vi "trim_space.vi"(1 "string in":string) -> (0 "string out":string)   [LabVIEW 2011]
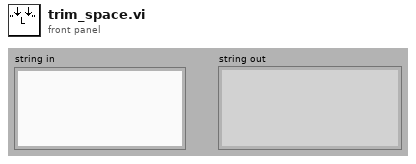
[diagram p1: front panel]
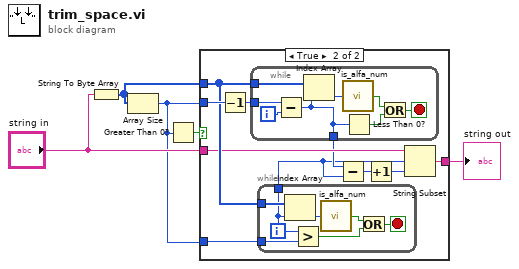
[diagram p0: block diagram]
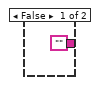
[diagram p2: hidden frame]
diagram:
  n1 = String To Byte Array(string="string in") -> (unsigned byte array=w3:u8[])
  n2 = Array Size(array=w3) -> (size(s)=w1:i32)
  n3 = Greater Than 0?(x=w1) -> (x > 0?=w2:bool)
  n4 = case shown="True" w2 {
    tunnel: ["" ("string in") w16] -> w5
    tunnel: w1 -> [_ w15]
    tunnel: w3 -> [_ w13]
    tunnel: "string in" -> [_ w12]
    tunnel: w1 -> [_ w7]
    frame False {
    }
    frame True {
      n5 = Decrement(x=w15) -> (x-1=w14:i32)
      n6 = while {
        tunnel: w13 -> [w24]
        tunnel: w14 -> [w22]
        tunnel: [w20] -> w11
        i -> [w21]
        stop <- w17 stop-if-true
        n7 = Subtract(x=w22, y=w21) -> (x-y=w20:i32)
        n8 = Index Array(array=w24, index=w20) -> (element=w23:u8)
        n9 = call "is_alfa_num.vi"("char"=w23) -> ("isAlfaNum"=w18:bool)
        n10 = Less Than 0?(x=w20) -> (x < 0?=w19:bool)
        n11 = Or(x=w18, y=w19) -> (x .or. y?=w17:bool)
      }
      n12 = while {
        tunnel: w13 -> [w31]
        tunnel: [w29] -> w10
        tunnel: w7 -> [w28]
        i -> [w29]
        stop <- w25 stop-if-true
        n13 = Index Array(array=w31, index=w29) -> (element=w30:u8)
        n14 = Greater?(x=w29, y=w28) -> (0:w26:bool)
        n15 = call "is_alfa_num.vi"("char"=w30) -> ("isAlfaNum"=w27:bool)
        n16 = Or(x=w27, y=w26) -> (x .or. y?=w25:bool)
      }
      n17 = Subtract(x=w11, y=w10) -> (x-y=w9:i32)
      n18 = Increment(x=w9) -> (x+1=w8:i32)
      n19 = String Subset(string=w12, offset (0)=w10, length (rest)=w8) -> (substring=w16:string)
    }
  }
  "string out" <- w5
